vi "GetTunnels.vi"(6 "error in":errorcluster, 9 "ForLoop in":refnum<class "ForLoop.lvclass">) -> (0 "error out":errorcluster, 3 "ForLoop out":refnum<class "ForLoop.lvclass">, 4 "Tunnels":i32[](array[numeric]))   [LabVIEW 2014]
uses:
  ForLoop.lvclass
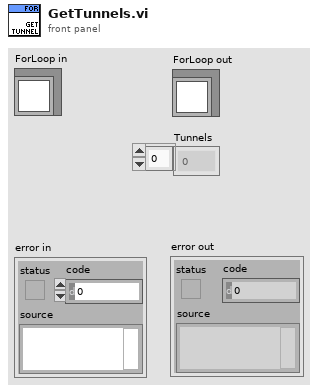
[diagram p1: front panel]
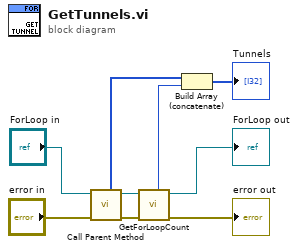
[diagram p0: block diagram]
diagram:
  n1 = call-parent "Call Parent Method"("error in"="error in", "Loop in"="ForLoop in") -> ("error out"=w4:errorcluster, "Loop out"=w6:refnum<class "ForLoop.lvclass">, "Tunnels"=w9:i32[])  [unwired: 5 in]
  n2 = call-dynamic "GetForLoopCount.vi"("error in"=w4, "ForLoop in"=w6) -> ("error out"=→"error out":errorcluster, "ForLoop out"=→"ForLoop out":refnum<class "ForLoop.lvclass">, "count UID"=w1:i32)  [unwired: 5 in]
  n3 = Build Array (concatenate)(w9, w1) -> (→"Tunnels":i32[])
